vi "Copy Image to Memory Address (ARGB).vi"(8 "error in (no error)":errorcluster, 10 "Destination":T2, 11 "ARGB Image Source":T1) -> (0 "error out":errorcluster, 3 "Destination (Duplcate)":T2)   [LabVIEW 2020, in "g_ar_toolkit.image.lvlib"]
uses:
  g_ar_toolkit.image.lvlib
  Raw Memory Information.ctl
  Raw Memory Information Dimension.ctl
  ARGB Image.ctl
  01eda17f-9221-4e43-bf47-cf9d986167a3.vi
  g_ar_toolkit.common/Module Path.vi
  <vilib>/Utility/error.llb/Error Cluster From Error Code.vi
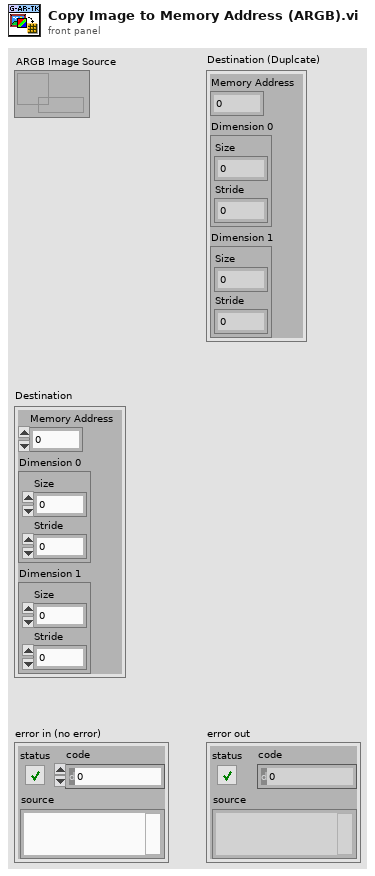
[diagram p1: front panel]
types:
  T1 = typedef "g_ar_toolkit.image.lvlib/ARGB Image.ctl" = refnum<data-value>
  T2 = typedef "g_ar_toolkit.image.lvlib/Raw Memory Information.ctl" = cluster{"Memory Address":u64, "Dimension 0":T3, "Dimension 1":T3}
  T3 = typedef "g_ar_toolkit.image.lvlib/Raw Memory Information Dimension.ctl" = cluster{"Size":u16, "Stride":u32}
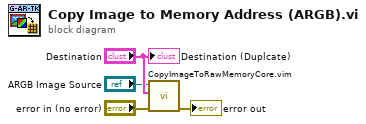
[diagram p0: block diagram]
diagram:
  n1 = call "CopyImageToRawMemoryCore.vim"("error in (no error)"="error in (no error)", "Destination"="Destination", "Src"="ARGB Image Source") -> ("error out"=→"error out":errorcluster)  [unwired: 8 in]
  "Destination (Duplcate)" <- "Destination"
